vi "Pass If Equal 1D Array (Numeric).vi"(6 "delta (optional)":ext, 8 "error in (no error)":errorcluster, 9 "actual":ext[](array[numeric]), 10 "expected":ext[](array[numeric]), 11 "TestCase in":refnum<class "TestCase.lvclass">) -> (0 "error out":errorcluster, 3 "TestCase out":refnum<class "TestCase.lvclass">)   [LabVIEW 2015, in "VITAC.lvlib"]
doc: "Compares two 1D numeric arrays and returns a pass/fail if any elements exceed the provided delta value (default = 0)\n\nThe results string will identify the numbers that don't match as well as the array index.\n\nThe VI takes EXT but has been tested to work with coerced SGL, DBL and integers."
uses:
  VITAC.lvlib
  <vilib>/addons/_JKI Toolkits/VI Tester/TestCase.llb/TestCase.lvclass
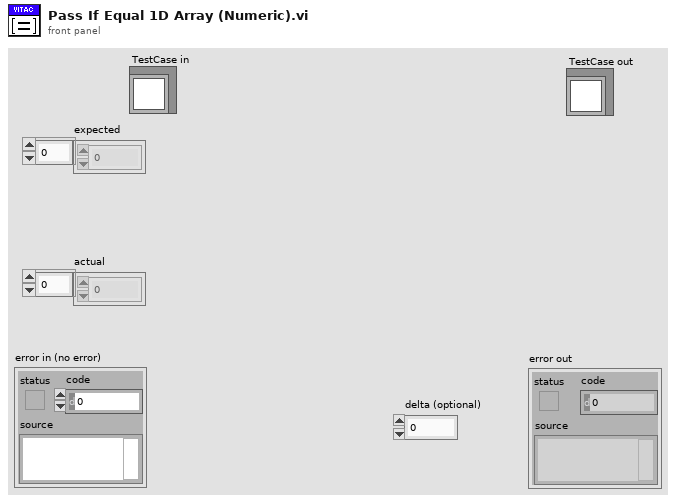
[diagram p1: front panel]
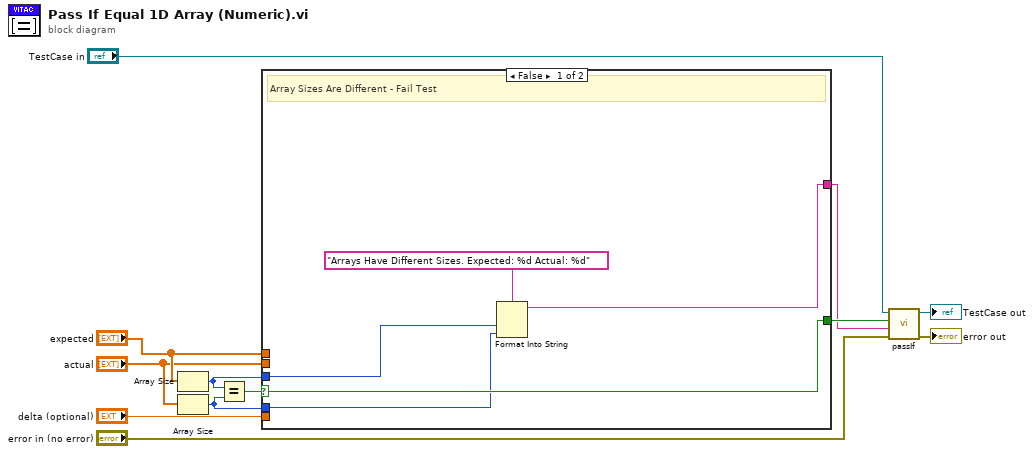
[diagram p0: block diagram]
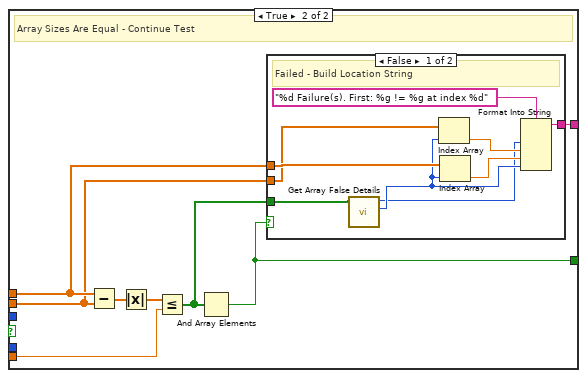
[diagram p2: hidden frame]
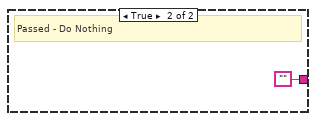
[diagram p3: hidden frame]
diagram:
  n1 = Array Size(array="expected") -> (size(s)=w2:i32)
  n2 = Array Size(array="actual") -> (size(s)=w1:i32)
  n3 = Equal?(x=w2, y=w1) -> (x = y?=w3:bool)
  n4 = case shown="False" w3 {
    selector: w3 -> [w17 _]
    tunnel: "delta (optional)" -> [_ w23]
    tunnel: [w17 w22] -> w7
    tunnel: [w13 w20] -> w6
    tunnel: "expected" -> [_ w19]
    tunnel: "actual" -> [_ w18]
    tunnel: w2 -> [w14 _]
    tunnel: w1 -> [w15 _]
    frame False {
      # "Array Sizes Are Different - Fail Test"
      n5 = Format Into String(format string="Arrays Have Different Sizes. Expected: %d Actual: %d", w14, w15) -> (resulting string=w13:string)  [unwired: 2 in, 1 out]
    }
    frame True {
      # "Array Sizes Are Equal - Continue Test"
      n6 = Subtract(x=w19, y=w18) -> (x-y=w25:ext[])
      n7 = Absolute Value(x=w25) -> (abs(x)=w24:ext[])
      n8 = Less Or Equal?(x=w24, y=w23) -> (x <= y?=w21:bool[])
      n9 = And Array Elements(Boolean array=w21) -> (logical AND=w22:bool)
      n10 = case shown="False" w22 {
        tunnel: w21 -> [w28 _]
        tunnel: w19 -> [w30 _]
        tunnel: w18 -> [w29 _]
        tunnel: [w31 ""] -> w20
        frame False {
          # "Failed - Build Location String"
          n11 = call "Get Array False Details.vi"("Array"=w28) -> ("First False"=w27:i32, "Count"=w26:i16)  [unwired: 9 in]
          n12 = Index Array(array=w29, index=w27) -> (element=w33:ext)
          n13 = Index Array(array=w30, index=w27) -> (element=w32:ext)
          n14 = Format Into String(format string="%d Failure(s). First: %g != %g at index %d", w26, w33, w32, w27) -> (resulting string=w31:string)  [unwired: 2 in, 1 out]
        }
        frame True {
          # "Passed - Do Nothing"
        }
      }
    }
  }
  n15 = call-dynamic "passIf.vi"("error in (no error)"="error in (no error)", "message (\"\")"=w6, "pass"=w7, "TestCase in"="TestCase in") -> ("error out"=→"error out":errorcluster, "TestCase out"=→"TestCase out":refnum<class "TestCase.lvclass">)  [unwired: 6 in]
